vi "Degrees To Radians.vi"(11 "Angle (°)":sgl) -> (3 "Angle (rad)":sgl)   [LabVIEW 2020, in "3D (FPGA).lvlib"]
uses:
  3D (FPGA).lvlib
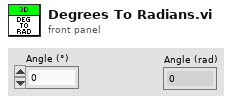
[diagram p1: front panel]
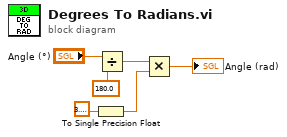
[diagram p0: block diagram]
diagram:
  n1 = To Single Precision Float(number=3.141592653589793) -> (single precision float=w2:sgl)
  n2 = Divide(x="Angle (°)", y=sgl 180.0) -> (x/y=w4:sgl)
  n3 = Multiply(x=w4, y=w2) -> (x*y=→"Angle (rad)":sgl)
